vi "ModbusLabView.vi"() -> ()   [LabVIEW 2015]
uses:
  <vilib>/NI Modbus.llb/MB Serial Master Query Read Coils (poly).vi
  <vilib>/NI Modbus.llb/MB Serial Master Query Write Multiple Coils (poly).vi
panel:
  in  "D0":bool[](array[boolean])
  in  "Starting Address 2":dbl
  in  "Cluster 2":cluster{"Slave Address":dbl, "Mode":i64}
  out "Exception Code 2":i16
  in  "Mode 2":i8
  in  "VISA 2":string(combo)
  out "Coils":bool[](array[boolean])
  out "Exception Code":i16
  in  "Cluster":cluster{"Slave Address":dbl, "Mode":i64}
  in  "VISA":string(combo)
  in  "Mode":i8
  in  "Starting Address":dbl
  in  "Quantity":dbl
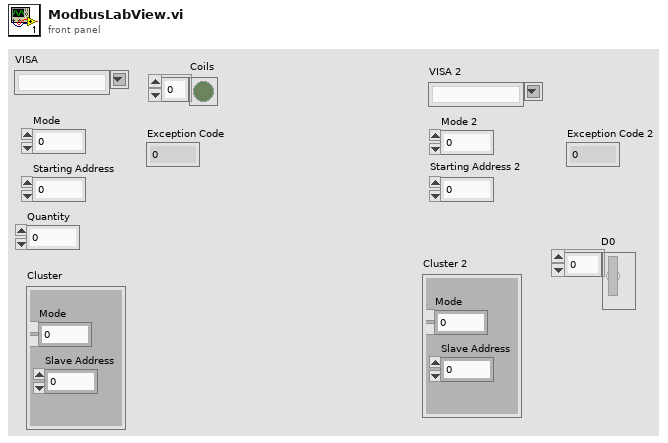
[diagram p1: front panel]
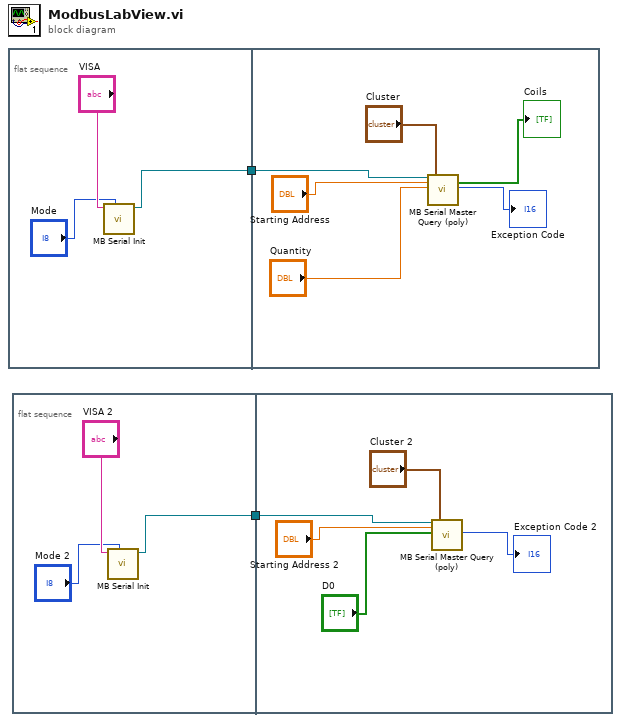
[diagram p0: block diagram]
diagram:
  n1 = flat-sequence {
    tunnel: [w4] -> w2
    tunnel: w2 -> [w9]
    frame #0 {
      n2 = call <vilib>:"MB Serial Init.vi"("Mode"="Mode", "VISA resource name"="VISA") -> ("VISA resource name out"=w4:refnum<visa-resource-name>)  [unwired: 8 in, 1 out]
    }
    frame #1 {
      n3 = call-poly <vilib>:"MB Serial Master Query (poly).vi"("VISA resource name"=w9, "Starting Address"="Starting Address", "Quantity"="Quantity", "Serial Parameters"="Cluster") -> ("Coils"=→"Coils":bool[], "Exception Code"=→"Exception Code":u8)  [unwired: 12 in, 2 out]
    }
  }
  n4 = flat-sequence {
    tunnel: [w13] -> w1
    tunnel: w1 -> [w18]
    frame #0 {
      n5 = call <vilib>:"MB Serial Init.vi"("Mode"="Mode 2", "VISA resource name"="VISA 2") -> ("VISA resource name out"=w13:refnum<visa-resource-name>)  [unwired: 8 in, 1 out]
    }
    frame #1 {
      n6 = call-poly <vilib>:"MB Serial Master Query (poly).vi"("VISA resource name"=w18, "Starting Address"="Starting Address 2", "Coils"="D0", "Serial Parameters"="Cluster 2") -> ("Exception Code"=→"Exception Code 2":u8)  [unwired: 13 in, 2 out]
    }
  }
